vi "Set CPU FFT Config.vi"(8 "error in (no error)":errorcluster, 10 "CPU FFT Size":u64=2000000 format="%.0p Samples", 11 "Application Manager in":refnum<class "Application Manager.lvclass">) -> (0 "error out":errorcluster, 3 "Application Manager out":refnum<class "Application Manager.lvclass">)   [LabVIEW 2020, in "Application Manager.lvlib" / "Application Manager.lvclass"]
uses:
  Application Manager.lvclass
  Application Manager.lvclass/Application Manager.ctl
  CPU FFT Calculator/CPU FFT Calculator Messages/Set FFT Config Msg/Set FFT Config Msg.lvclass/Set FFT Config Msg.ctl
  <vilib>/ActorFramework/Message Enqueuer/Message Enqueuer.lvclass/Message Enqueuer.ctl
  <vilib>/ActorFramework/Message Enqueuer/Enqueue.vi
  CPU FFT Calculator/CPU FFT Calculator Messages/Set FFT Config Msg/Set FFT Config Msg.lvclass
  C:/Program Files/National Instruments/LabVIEW 2026/vi.lib/ActorFramework/Message/Message.lvclass
  <vilib>/ActorFramework/Message Priority Queue/Priority Enqueue.vi
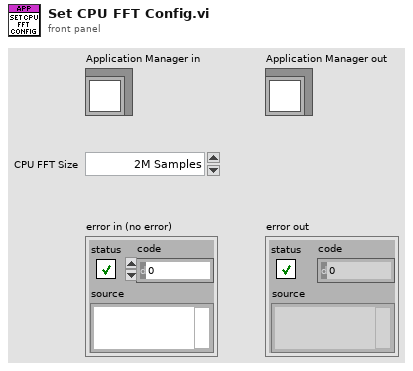
[diagram p1: front panel]
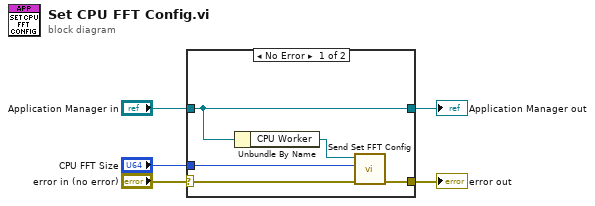
[diagram p0: block diagram]
diagram:
  n1 = case shown="No Error" "error in (no error)" {
    selector: "error in (no error)" -> [w10 w12]
    tunnel: [w9 w12] -> w4
    tunnel: [w7 w11] -> w2
    tunnel: "Application Manager in" -> [w7 w11]
    tunnel: "CPU FFT Size" -> [w8 _]
    frame No Error {
      n2 = Unbundle By Name(w7) -> ("CPU Worker"=w6:refnum<class "Message Enqueuer.lvclass">)
      n3 = call "Send Set FFT Config.vi"("error in (no error)"=w10, "CPU FFT Size"=w8, "Message Enqueuer"=w6) -> ("error out"=w9:errorcluster)  [unwired: 7 in, 1 out]
    }
    frame Error {
    }
  }
  "error out" <- w4
  "Application Manager out" <- w2
